vi "Hold Edge.vi"(0 "Trigger":bool, 1 "Reset?":bool) -> (2 "Signal?":bool)   [LabVIEW 2021]
doc: "The <b>Signal?</b> Boolean changes to TRUE when a rising edge is detected on the <b>Trigger</b> input. The <b>Signal?</b> Boolean remains TRUE unless the <b>Reset?</b> line is held high."
panel:
  # "The Signal? Boolean changes to TRUE when a rising edge is detected on the Trigger input. The Signal? Boolean remains TRUE unless the Reset? line is held high."
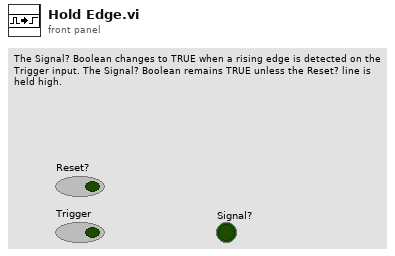
[diagram p1: front panel]
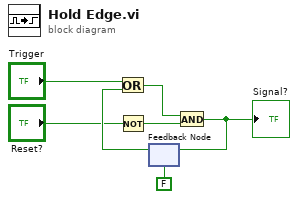
[diagram p0: block diagram]
diagram:
  n1 = Not(x="Reset?") -> (.not. x?=w3:bool)
  n2 = feedback #1(FALSE) -> (w7:bool)
  n3 = Or(x="Trigger", y=w7) -> (x .or. y?=w5:bool)
  n4 = And(x=w5, y=w3) -> (x .and. y?=w4:bool)
  "Signal?" <- w4
  n5 = feedback-in #1(w4) -> ()
